vi "GetChamber.vi"(6 "error in (no error)":errorcluster, 7 "Instrument Ref In":refnum<k24>) -> (0 "GetChamber Error":i32, 1 "Chamber\nStatus":i32(ring) items=["ChamberUnknown"=0, "PurgedAndSealed"=1, "VentedAndSealed"=2, "Sealed"=3, "Purging"=4, "Venting"=5, "PreHiVac"=6, "HighVac"=7, "PumpContinuous"=8, "VentContinuous"=9, "ChamberFailure"=15], 2 "error out":errorcluster, 3 "Instrument Ref Out":refnum<k24>)   [LabVIEW 2016]
uses:
  C:/user/patrick/hg/levylab_inst_ppms2/lvsrc/PPMS2/QDInstrument_LabView/QDInstrument.dll
  PPMS2/QDInstrument_LabView/QDInstrument.dll
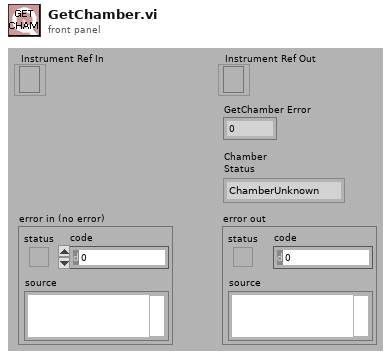
[diagram p1: front panel]
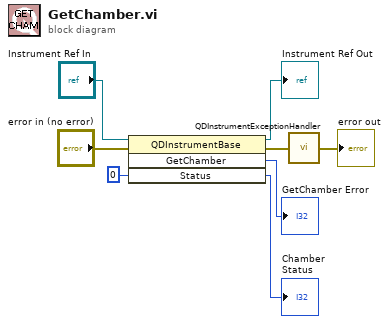
[diagram p0: block diagram]
diagram:
  n1 = invoke class="QDInstrumentBase" method="GetChamber"(reference="Instrument Ref In", error in="error in (no error)", "Status"=0) -> (reference out=→"Instrument Ref Out":refnum<k24>, error out=w2:errorcluster, "GetChamber"=→"GetChamber Error":i32, "Status"=→"Chamber\nStatus":i32)  [unwired: 1 in]
  n2 = call "QDInstrumentExceptionHandler.vi"("Error in"=w2) -> ("Error out"=→"error out":errorcluster)
